vi "MUX Testing_v2 - Copy.vi"() -> ()   [LabVIEW 2011]
uses:
  <vilib>/ULx/Create Channel.llb/ULx Create Channel (DO-Digital Output).vi
  <vilib>/ULx/Write.llb/ULx Write (Digital U32 1Chan 1Samp).vi
panel:
  in  "Port":refnum<k21>="Dev0/AuxPort"
  # "WATCH THE LEDS!"
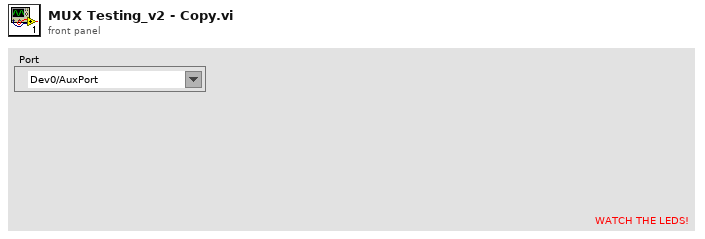
[diagram p1: front panel]
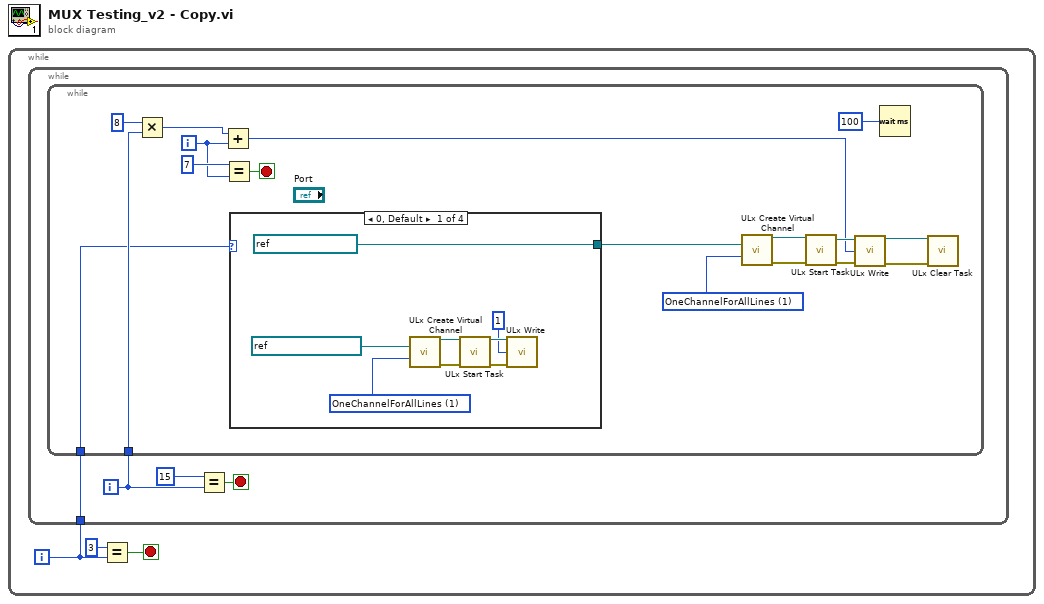
[diagram p0: block diagram]
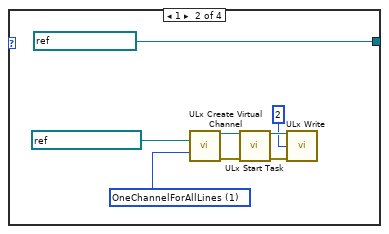
[diagram p2: hidden frame]
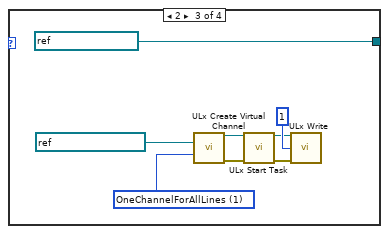
[diagram p3: hidden frame]
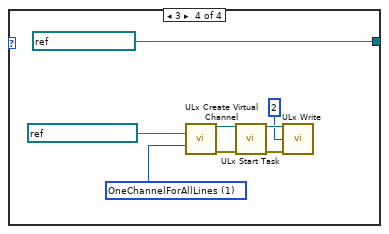
[diagram p4: hidden frame]
diagram:
  n1 = while {
    i -> [w1]
    stop <- w2 stop-if-true
    n2 = while {
      tunnel: w1 -> [w4]
      i -> [w7]
      stop <- w5 stop-if-true
      n3 = while {
        tunnel: w7 -> [w10]
        tunnel: w4 -> [w9]
        i -> [w12]
        stop <- w11 stop-if-true
        w23 = 1 items=["OneChannelForEachLine", "OneChannelForAllLines"] ("line grouping")
        n4 = Multiply(x=8, y=w10) -> (x*y=w15:i32)
        n5 = Add(x=w15, y=w12) -> (x+y=w14:i32)
        n6 = Equal?(x=7, y=w12) -> (x = y?=w11:bool)
        n7 = case shown="0, Default" w9 {
          tunnel: [refnum<k21> "Dev0/1stPortA" ("Port 2") refnum<k21> "Dev0/1stPortB" ("Port 2") refnum<k21> "Dev1/1stPortA" ("Port 2") refnum<k21> "Dev1/1stPortB" ("Port 2")] -> w24
          frame 0, Default {
            w31 = 1 items=["OneChannelForEachLine", "OneChannelForAllLines"] ("line grouping")
            n8 = call-poly <vilib>:"ULx Create Virtual Channel.vi"("lines"=refnum<k21> "Dev0/1stPortCL" ("Port 2"), "line grouping"=w31) -> ("task out"=w28:refnum<k24>, "error out"=w27:errorcluster)  [unwired: 12 in]
            n9 = call <vilib>:"ULx Start Task.vi"("task in"=w28, "error in"=w27) -> ("task out"=w29:refnum<k24>, "error out"=w30:errorcluster)  [unwired: 12 in]
            n10 = call-poly <vilib>:"ULx Write.vi"("task in"=w29, "data"=1, "error in"=w30) -> ()  [unwired: 10 in, 3 out]
          }
          frame 1 {
            w39 = 1 items=["OneChannelForEachLine", "OneChannelForAllLines"] ("line grouping")
            n11 = call-poly <vilib>:"ULx Create Virtual Channel.vi"("lines"=refnum<k21> "Dev0/1stPortCL" ("Port 2"), "line grouping"=w39) -> ("task out"=w36:refnum<k24>, "error out"=w35:errorcluster)  [unwired: 12 in]
            n12 = call <vilib>:"ULx Start Task.vi"("task in"=w36, "error in"=w35) -> ("task out"=w37:refnum<k24>, "error out"=w38:errorcluster)  [unwired: 12 in]
            n13 = call-poly <vilib>:"ULx Write.vi"("task in"=w37, "data"=2, "error in"=w38) -> ()  [unwired: 10 in, 3 out]
          }
          frame 2 {
            w41 = 1 items=["OneChannelForEachLine", "OneChannelForAllLines"] ("line grouping")
            n14 = call-poly <vilib>:"ULx Create Virtual Channel.vi"("lines"=refnum<k21> "Dev1/1stPortCL" ("Port 2"), "line grouping"=w41) -> ("task out"=w44:refnum<k24>, "error out"=w45:errorcluster)  [unwired: 12 in]
            n15 = call <vilib>:"ULx Start Task.vi"("task in"=w44, "error in"=w45) -> ("task out"=w43:refnum<k24>, "error out"=w42:errorcluster)  [unwired: 12 in]
            n16 = call-poly <vilib>:"ULx Write.vi"("task in"=w43, "data"=1, "error in"=w42) -> ()  [unwired: 10 in, 3 out]
          }
          frame 3 {
            w55 = 1 items=["OneChannelForEachLine", "OneChannelForAllLines"] ("line grouping")
            n17 = call-poly <vilib>:"ULx Create Virtual Channel.vi"("lines"=refnum<k21> "Dev1/1stPortCL" ("Port 2"), "line grouping"=w55) -> ("task out"=w52:refnum<k24>, "error out"=w51:errorcluster)  [unwired: 12 in]
            n18 = call <vilib>:"ULx Start Task.vi"("task in"=w52, "error in"=w51) -> ("task out"=w53:refnum<k24>, "error out"=w54:errorcluster)  [unwired: 12 in]
            n19 = call-poly <vilib>:"ULx Write.vi"("task in"=w53, "data"=2, "error in"=w54) -> ()  [unwired: 10 in, 3 out]
          }
        }
        n20 = call-poly <vilib>:"ULx Create Virtual Channel.vi"("lines"=w24, "line grouping"=w23) -> ("task out"=w21:refnum<k24>, "error out"=w22:errorcluster)  [unwired: 12 in]
        n21 = call <vilib>:"ULx Start Task.vi"("task in"=w21, "error in"=w22) -> ("task out"=w18:refnum<k24>, "error out"=w17:errorcluster)  [unwired: 12 in]
        n22 = call-poly <vilib>:"ULx Write.vi"("task in"=w18, "data"=w14, "error in"=w17) -> ("task out"=w20:refnum<k24>, "error out"=w19:errorcluster)  [unwired: 10 in, 1 out]
        n23 = Wait (ms)(milliseconds to wait=100) -> ()  [unwired: 1 out]
        n24 = call <vilib>:"ULx Clear Task.vi"("task in"=w20, "error in"=w19) -> ()  [unwired: 13 in, 1 out]
      }
      n25 = Equal?(x=15, y=w7) -> (x = y?=w5:bool)
    }
    n26 = Equal?(x=3, y=w1) -> (x = y?=w2:bool)
  }
